vi "MainGlobalConstants.vi"() -> ()   [LabVIEW 2010]
panel:
  in  "Sub VI Refnum":refnum<vi>
  out "EXIT":bool
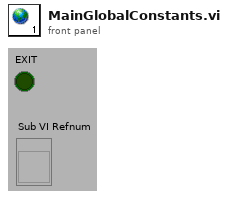
[diagram p1: front panel]
diagram:
